vi "CreateBusChannel.vi"(9 "1st child channel index":i32, 10 "Bus Name":string, 11 "Wfm Data in":waveform(sgl)[](array[waveform])) -> (1 "Created Bus Channel":waveform(sgl), 3 "Wfm Data out":waveform(sgl)[](array[waveform]))   [LabVIEW 2017, in "McsaVirtualChannel.lvlib"]
uses:
  <vilib>/addons/InsightCM/Devices/Shared/Mcsa/McsaVirtualChannel/McsaVirtualChannel.lvlib
  <vilib>/addons/InsightCM/Utilities/ChannelStatus/ChannelStatus.lvlib
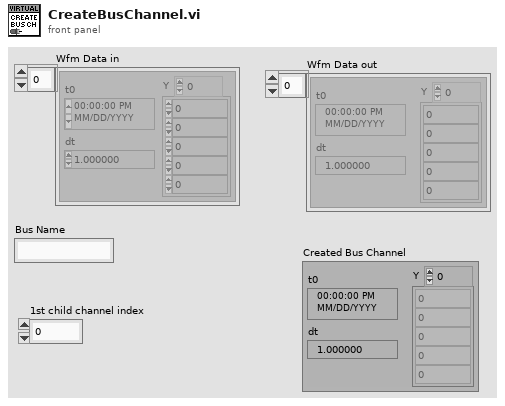
[diagram p1: front panel]
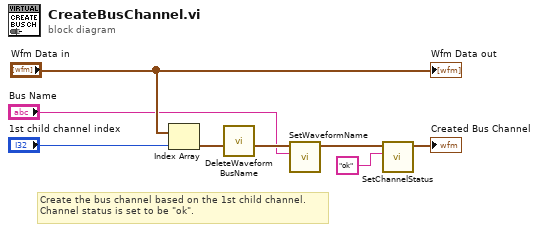
[diagram p0: block diagram]
diagram:
  # "Create the bus channel based on the 1st child channel.\nChannel status is set to be \"ok\"."
  n1 = Index Array(array="Wfm Data in", index="1st child channel index") -> (element=w6:waveform(sgl))
  n2 = call <vilib>:"DeleteWaveformBusName.vi"("Waveform in"=w6) -> ("Waveform out"=w3:waveform(sgl))  [unwired: 9 in, 1 out]
  n3 = call <vilib>:"SetWaveformName.vi"("Name"="Bus Name", "Waveform in"=w3) -> ("Waveform out"=w1:waveform(sgl))  [unwired: 8 in, 1 out]
  n4 = call <vilib>:"SetChannelStatus.vi"("Channel Status"="ok", "Waveform in"=w1) -> ("Waveform out"=→"Created Bus Channel":waveform(sgl))  [unwired: 8 in, 1 out]
  "Wfm Data out" <- "Wfm Data in"
